vi "LvMPDC_CMD_playlist.vi"(6 "timeout_ms":i32=25000, 8 "error in (no error)":errorcluster, 9 "ReadBytes":i32=1024, 11 "Connect ID":refnum<k5>) -> (0 "error out":errorcluster, 1 "playlist path[]":path[](array[path]), 3 "Connect ID out":refnum<k5>)   [LabVIEW 2012]
panel:
  # "LvMPDC:: CMD playlist"
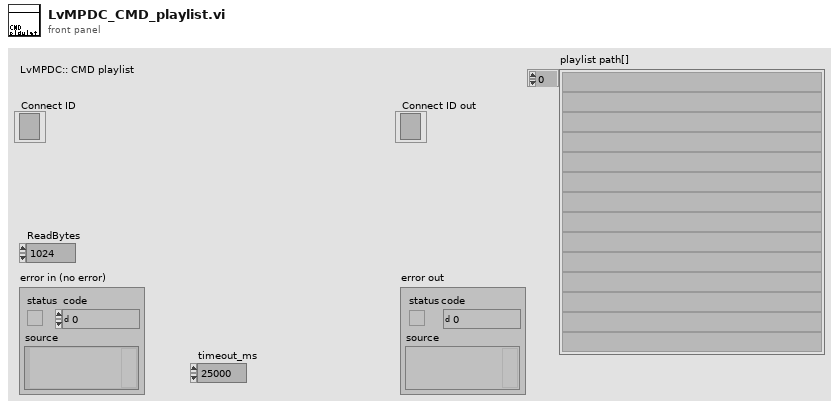
[diagram p1: front panel]
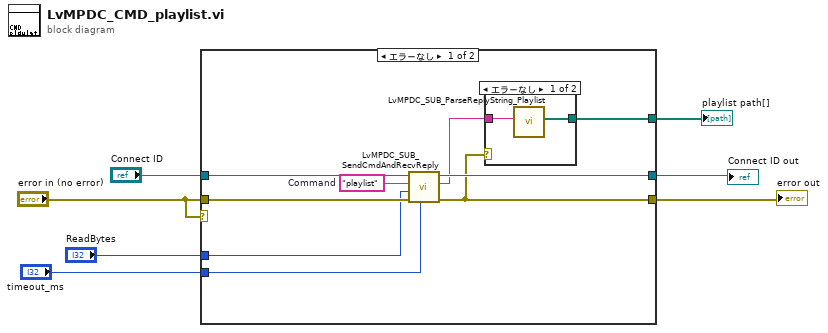
[diagram p0: block diagram]
diagram:
  n1 = case shown="エラーなし" "error in (no error)" {
    tunnel: "Connect ID" -> [w15 w20]
    tunnel: "error in (no error)" -> [w16 w19]
    tunnel: [w14 w20] -> w6
    tunnel: [w10 w19] -> w5
    tunnel: "timeout_ms" -> [w11 _]
    tunnel: "ReadBytes" -> [w12 _]
    tunnel: [w8 _] -> w1
    frame No Error {
      w13 = "playlist"  # Command
      n2 = call "LvMPDC_SUB_SendCmdAndRecvReply.vi"("timeout_ms"=w11, "error in (no error)"=w16, "ReadBytes"=w12, "Command"=w13, "Connect ID"=w15) -> ("error out"=w10:errorcluster, "Reply"=w9:string, "Connect ID out"=w14:refnum<k5>)  [unwired: 4 in]
      n3 = case shown="エラーなし" w10 {
        tunnel: w9 -> [w18 _]
        tunnel: [w17 _] -> w8
        frame No Error {
          n4 = call "LvMPDC_SUB_ParseReplyString_Playlist.vi"("string"=w18) -> ("playlist path[]"=w17:path[])  [unwired: 10 in]
        }
        frame Error {
        }
      }
    }
    frame Error {
    }
  }
  "Connect ID out" <- w6
  "error out" <- w5
  "playlist path[]" <- w1
